vi "FTW-ERR-ThrowGenericError.vi"(7 "Error Message":string, 11 "error in":errorcluster) -> (15 "error out":errorcluster)   [LabVIEW 2014]
panel:
  # "Inputs"
  # "Outputs"
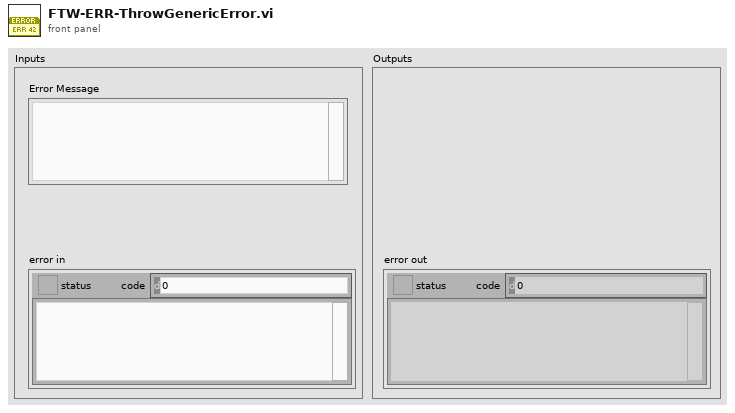
[diagram p1: front panel]
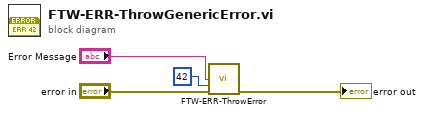
[diagram p0: block diagram]
diagram:
  n1 = call "FTW-ERR-ThrowError.vi"("Error Message"="Error Message", "Error Code"=42 ("code"), "error in"="error in") -> ("error out"=→"error out":errorcluster)  [unwired: 12 in]
